vi "clearAll.vi"(8 "error in (no error)":errorcluster, 11 "CompiledList in":refnum<class "CompiledList.lvclass">) -> (0 "error out":errorcluster, 3 "CompiledList out":refnum<class "CompiledList.lvclass">)   [LabVIEW 2011, in "Compiler.lvlib" / "CompiledList.lvclass"]
uses:
  CompiledList.lvclass
  ScriptListCompiler/ScriptListCompiler.lvclass
  Hal/Channels/VoltOutput/AnalogOutput.lvclass
  Hal/Channels/Digital/DigitalOutput.lvclass
  Hal/Channels/DDSOutput/Generic/DDSOutput.lvclass
  CompiledList.lvclass/CompiledList.ctl
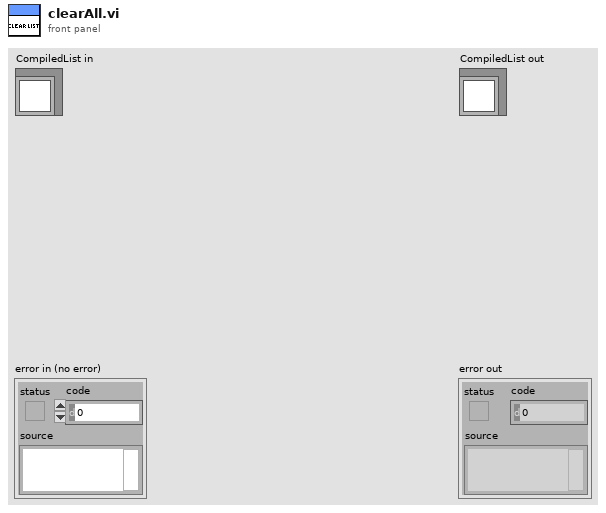
[diagram p1: front panel]
types:
  T1 = cluster{"ScriptListCompiler.lvclass":refnum<class "ScriptListCompiler.lvclass">, "aoChannels":refnum<class "AnalogOutput.lvclass">[], "doChannels":refnum<class "DigitalOutput.lvclass">[], "rfChannels":refnum<class "DDSOutput.lvclass">[]}[]
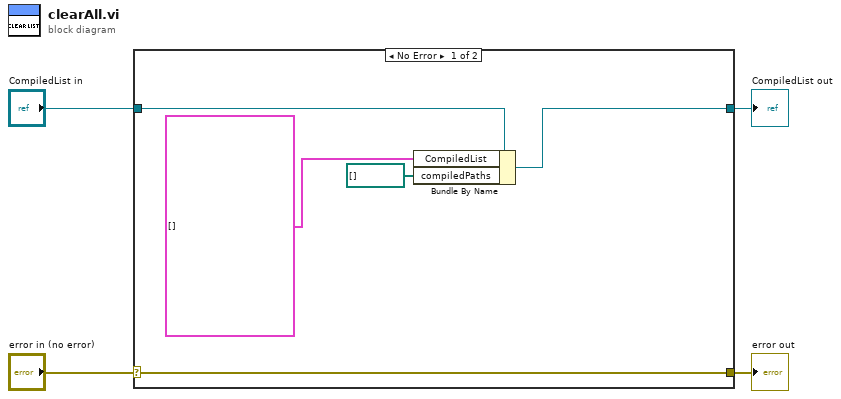
[diagram p0: block diagram]
diagram:
  n1 = case shown="No Error" "error in (no error)" {
    selector: "error in (no error)" -> [w9 w11]
    tunnel: [w9 w11] -> w3
    tunnel: [w7 w10] -> w1
    tunnel: "CompiledList in" -> [w8 w10]
    frame No Error {
      n2 = Bundle By Name(cluster=w8, "CompiledList"=T1 [], "compiledPaths"=path[] []) -> (w7:refnum<class "CompiledList.lvclass">)
    }
    frame Error {
    }
  }
  "error out" <- w3
  "CompiledList out" <- w1
